vi "indirectPathAngleV2.vi"() -> ()   [LabVIEW 2017]
uses:
  <vilib>/imath/engines/lvmath2/RunTimeEngine/Managers/WorkSpace/UID Generator.vi
  <vilib>/imath/engines/lvmath2/RunTimeEngine/IndexRead/NIMS V(S).vi
  <instcachedir>/0/NIMS V(S)_0488751826AF41519A22953C041130DC.lvgen/NIMS V(S)_0488751826AF41519A22953C041130DC_000.vi
  <vilib>/imath/engines/lvmath2/RunTimeEngine/BuiltInFunctions/abs/NIMS_abs(signed).vi
  <instcachedir>/0/NIMS_abs(signed)_C4FCB8E6058B49B797C7C8D53CA5F6EC.lvgen/NIMS_abs(signed)_C4FCB8E6058B49B797C7C8D53CA5F6EC_000.vi
  <vilib>/imath/engines/lvmath2/RunTimeEngine/RunTimeType/NIMS_RunTimeType_From StrictType (excl LVString).vi
  <instcachedir>/0/NIMS_RunTimeType_From StrictType (excl LVString)_1019F277F0A747EDBCA0F6C52CA54500.lvgen/NIMS_RunTimeType_From StrictType (excl LVString)_1019F277F0A747EDBCA0F6C52CA54500_000.vi
  <vilib>/imath/engines/lvmath2/RunTimeEngine/ErrorHandling/NIMS_Create Error From Enums.vi
  <vilib>/imath/engines/lvmath2/RunTimeEngine/LocalVariableDefStatement/MC_LocalVariableDefStatement_Display.vi
  <vilib>/imath/engines/lvmath2/RunTimeEngine/BuiltInFunctions/mirrorh/NIMS_mirrorh(GRowV).vi
  <instcachedir>/0/NIMS_mirrorh(GRowV)_B6A8CC4EAFBA4F9A82A59460D67BDFF0.lvgen/NIMS_mirrorh(GRowV)_B6A8CC4EAFBA4F9A82A59460D67BDFF0_001.vi
  <vilib>/imath/engines/lvmath2/RunTimeEngine/BuiltInFunctions/deg_to_rad/NIMS_deg_to_rad.vi
  <instcachedir>/0/NIMS_deg_to_rad_4A81D684CE8D4DD79924F5AB74D756E1.lvgen/NIMS_deg_to_rad_4A81D684CE8D4DD79924F5AB74D756E1_001.vi
  <vilib>/imathl/engines/lvmath/Functions/Error Handling/Create Error.vi
  <vilib>/imath/engines/lvmath2/RunTimeSupport/NIMS_Complex To Real.vi
  <instcachedir>/0/NIMS_Complex To Real_BE01396FDE034E8E94CEBBA1E368668D.lvgen/NIMS_Complex To Real_BE01396FDE034E8E94CEBBA1E368668D_001.vi
  <vilib>/imath/engines/lvmath2/RunTimeEngine/BuiltInFunctions/rad_to_deg/NIMS_rad_to_deg.vi
  <instcachedir>/0/NIMS_rad_to_deg_A39AFCDDC8C049FCADAAB7FC30B9F5AA.lvgen/NIMS_rad_to_deg_A39AFCDDC8C049FCADAAB7FC30B9F5AA_001.vi
  <vilib>/imath/engines/lvmath2/RunTimeEngine/Managers/SymbolTable/Clear UID.vi
  <vilib>/imath/engines/lvmath2/RunTimeEngine/NodeEndStatement/NIMS_NodeEndStatement_Output.vi
  <instcachedir>/0/NIMS_NodeEndStatement_Output_53EC0D466D134D7ABD903AC30B43404B.lvgen/NIMS_NodeEndStatement_Output_53EC0D466D134D7ABD903AC30B43404B_005.vi
  <instcachedir>/0/NIMS_NodeEndStatement_Output_53EC0D466D134D7ABD903AC30B43404B.lvgen/NIMS_NodeEndStatement_Output_53EC0D466D134D7ABD903AC30B43404B_001.vi
  <instcachedir>/0/NIMS_NodeEndStatement_Output_53EC0D466D134D7ABD903AC30B43404B.lvgen/NIMS_NodeEndStatement_Output_53EC0D466D134D7ABD903AC30B43404B_009.vi
  <vilib>/imath/engines/lvmath2/RunTimeEngine/ErrorHandling/NIMS_Finalize Error.vi
  <vilib>/imath/engines/lvmath2/RunTimeEngine/Managers/SymbolTable/NIMS_WorkSpace.lvlib
panel:
  out "pathAngles":dbl[](array[numeric])
  out "pathAngle":dbl
  out "lengthTerm2":dbl
  out "lengthTerm1":dbl
  out "interPathAngle":dbl
  out "angleB":dbl
  out "lengthC":dbl
  out "sorted path\nlengths":dbl[](array[numeric])
  out "sorted path\nangles":dbl[](array[numeric])
  out "component \npath angles":i32[](array[numeric])
  out "path axes":i32[](array[numeric])
  in  "goal platform":i32
  in  "start platform":i32
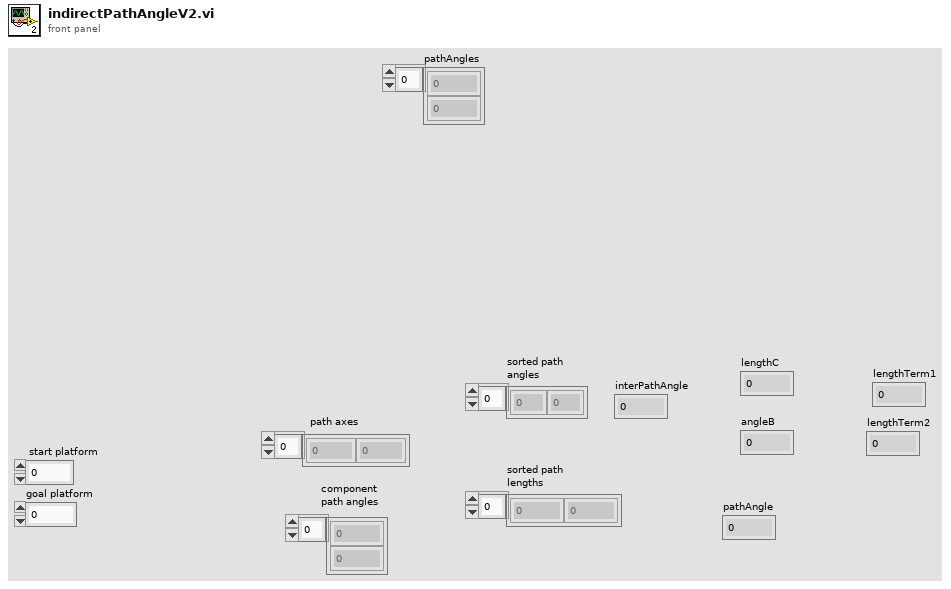
[diagram p1: front panel]
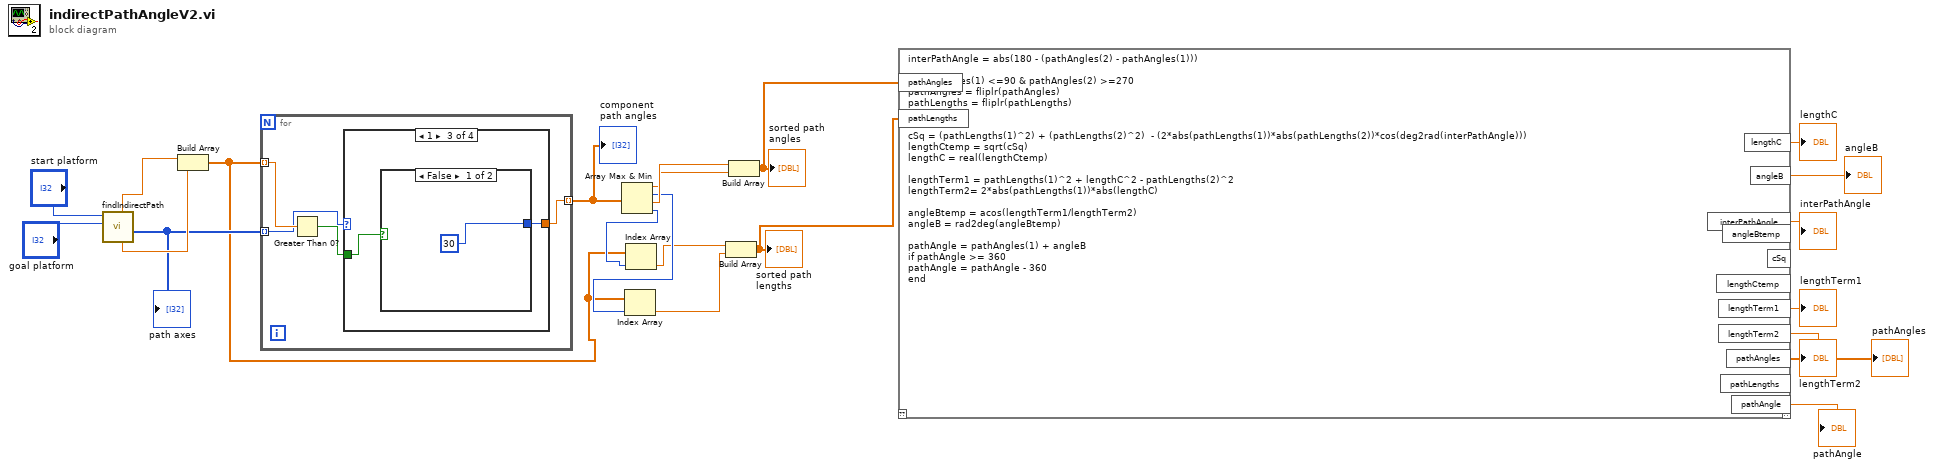
[diagram p0: block diagram]
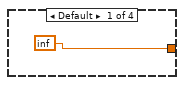
[diagram p2: hidden frame]
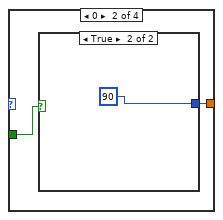
[diagram p3: hidden frame]
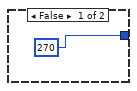
[diagram p4: hidden frame]
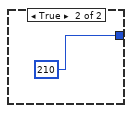
[diagram p5: hidden frame]
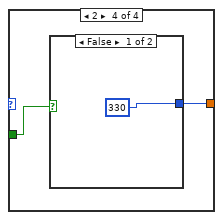
[diagram p6: hidden frame]
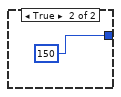
[diagram p7: hidden frame]
diagram:
  n1 = call "findIndirectPath.vi"("goal platform"="goal platform", "start platform"="start platform") -> ("path axes"=w13:i32[], "intersection to goal \ndistance"=w19:dbl, "start to intersection distance"=w20:dbl)  [unwired: 4 in, 3 out]
  "path axes" <- w13
  n2 = Build Array(w20, w19) -> (w10:dbl[])
  n3 = for {
    tunnel: w10 -> [w25] mode=indexing
    tunnel: w13 -> [w23] mode=indexing
    tunnel: [w26] -> w18 mode=indexing
    n4 = Greater Than 0?(x=w25) -> (x > 0?=w24:bool)
    n5 = case shown="1" w23 {
      tunnel: w24 -> [_ w29 w33 w37]
      tunnel: [inf w28 w32 w36] -> w26
      frame Default {
      }
      frame 0 {
        n6 = case shown="True" w29 {
          tunnel: [270 90] -> w28
          frame False {
          }
          frame True {
          }
        }
      }
      frame 1 {
        n7 = case shown="False" w33 {
          tunnel: [30 210] -> w32
          frame False {
          }
          frame True {
          }
        }
      }
      frame 2 {
        n8 = case shown="False" w37 {
          tunnel: [330 150] -> w36
          frame False {
          }
          frame True {
          }
        }
      }
    }
  }
  "component \npath angles" <- w18
  n9 = Array Max & Min(array=w18) -> (max value=w16:dbl, max index (indices)=w14:i32, min value=w17:dbl, min index (indices)=w15:i32)
  n10 = Index Array(array=w10, index=w14) -> (element=w11:dbl)
  n11 = Index Array(array=w10, index=w15) -> (element=w12:dbl)
  n12 = Build Array(w12, w11) -> (w8:dbl[])
  "sorted path\nlengths" <- w8
  n13 = Build Array(w17, w16) -> (w9:dbl[])
  "sorted path\nangles" <- w9
  n14 = mathscript code="interPathAngle = abs(180 - (pathAngles(2) - pathAngles(1)))\n\nif pathAngles(1) <=90 & pathAngles(2) >=270\npathAngles = fliplr(pathAngles)\npathLengths = fliplr(pathLengths)\nend\n\ncSq = (pathLengths(1)^2) + (pathLengths(2)^2)  - (2*abs(pathLengths(1))*abs(pathLengths(2))*cos(deg2rad(interPathAngle)))\nlengthCtemp = sqrt(cSq)\nlengthC = real(lengthCtemp)\n\nlengthTerm1 = pathLengths(1)^2 + lengthC^2 - pathLengths(2)^2\nlengthTerm2= 2*abs(pathLengths(1))*abs(lengthC)\n\nangleBtemp = acos(lengthTerm1/lengthTerm2)\nangleB = rad2deg(angleBtemp)\n\npathAngle = pathAngles(1) + angleB\nif pathAngle >= 360\npathAngle = pathAngle - 360\nend"("pathAngles"=w9, "pathLengths"=w8) -> ("lengthC"=→"lengthC":dbl, "angleB"=→"angleB":dbl, "interPathAngle"=→"interPathAngle":dbl, "lengthTerm1"=→"lengthTerm1":dbl, "lengthTerm2"=→"lengthTerm2":dbl, "pathAngles"=→"pathAngles":dbl[], "pathAngle"=→"pathAngle":dbl)  [unwired: 1 in, 5 out]
